vi "DSWrite uint32.vi"(8 "error in":errorcluster[](array[cluster]), 9 "ms timeout (10000)":i32, 10 "data":u32[](array[numeric]), 11 "connection in":refnum<k13>[](array[refnum])) -> (0 "error out":errorcluster[](array[cluster]), 3 "connection out":refnum<k13>[](array[refnum]))   [LabVIEW 2011]
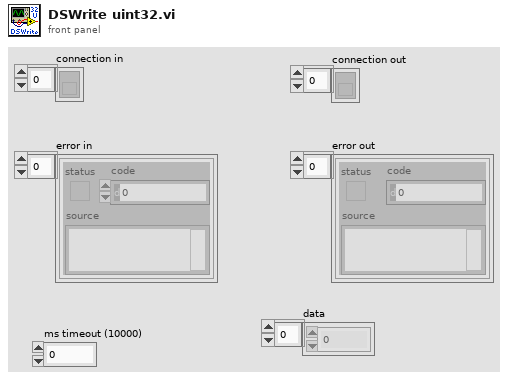
[diagram p1: front panel]
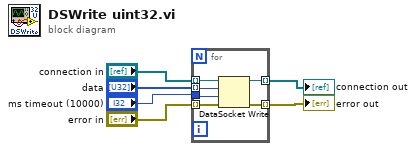
[diagram p0: block diagram]
diagram:
  n1 = for {
    tunnel: [w12] -> w3 mode=indexing
    tunnel: [w11] -> w4 mode=indexing
    tunnel: "connection in" -> [w10] mode=indexing
    tunnel: "error in" -> [w9] mode=indexing
    tunnel: "ms timeout (10000)" -> [w8]
    tunnel: "data" -> [w7] mode=indexing
    n2 = DataSocket Write(8:w9, 9:w8, 10:w7, 11:w10) -> (0:w12:errorcluster, 3:w11:refnum<k13>)  [unwired: 1 out]
  }
  "connection out" <- w4
  "error out" <- w3
